vi "Create Instance.vi"() -> (3 "PowerSupply_IT6333A.lvclass Out":refnum<class "PowerSupply_IT6333A.lvclass">)   [LabVIEW 2017, in "PowerSupply_IT6333A.lvclass"]
uses:
  PowerSupply_IT6333A.lvclass
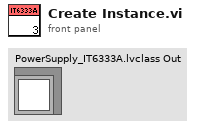
[diagram p1: front panel]
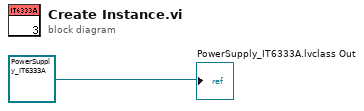
[diagram p0: block diagram]
diagram:
  "PowerSupply_IT6333A.lvclass Out" <- refnum<class "PowerSupply_IT6333A.lvclass"> refnum ("PowerSupply_IT6333A.lvclass")
